vi "RT_Control_Adrian_ForceBalance.vi"(11 "Parameters":T1={"N_chan"=0, "Input Rate (Hz)"=0.0, "Acq Time (s)"=0.0, "NumOfWarmupIters"=0, "Size fifo"=0, "Period NCL (ms)"=0, "Timeout fifo Read"=0, "Size Sent Array"=0, "Output offsets"=[], "Input offsets"=[0.0, 0.0, 0.0, 0.0, 0.0, 0.0, 0.0, 0.0]}) -> (0 "error out":errorcluster, 1 "Total Iterations":i64, 2 "Delayed Cycles":dbl)   [LabVIEW 2021]
uses:
  parametersRT.ctl
  <vilib>/DAQmx/write.llb/DAQmx Write (Analog 1D DBL NChan 1Samp).vi
  <vilib>/DAQmx/read.llb/DAQmx Read (Analog 1D DBL NChan 1Samp).vi
  <vilib>/Analysis/baseanly.llb/A x Vector.vi
  <vilib>/DAQmx/configure/timing.llb/DAQmx Timing (Sample Clock).vi
  <vilib>/DAQmx/miscellaneous.llb/DAQmx Fill In Error Info.vi
  <resource>/objmgr/daqmx.rc
  <vilib>/Analysis/NI_AALBase.lvlib
panel:
  in  "source 2":tag
  in  "source":tag
  out "coerced(x)":dbl[](array[numeric])
  out "A x Vector":dbl[](array[numeric]) format="%.2f"
  in  "Unbias":bool
  out "Bias Voltages":dbl[][](array[numeric])=[[-0.0710179470114859, -0.17463349299050945, -0.11016159714741332, 0.026018829634351103, 0.12897648926553976, 0.08259620236774425]]
  out "Bias Vector":dbl[](array[numeric])=[-0.0710179470114859, -0.17463349299050945, -0.11016159714741332, 0.026018829634351103, 0.12897648926553976, 0.08259620236774425]
  in  "Bias":bool
  out "Voltages":dbl[][](array[numeric])=[[-0.07200476171213811, -0.17430455474177844, -0.11114841186574954, 0.027005644288728526, 0.12535816905124034, 0.08062257311350753], [-0.07233369994578917, -0.17397561649309423, -0.11147735010529275, 0.027334582506747616, 0.1263449836558195, 0.08160938774087402], [-0.0716758234785372, -0.17463349299050945, -0.11147735010529275, 0.026676706070656076, 0.1260160454543497, 0.08062257311350753], [-0.07200476171213811, -0.1749624312392873, -0.1118062883448848, 0.026676706070656076, 0.1256871072528233, 0.08029363490427514], [-0.07200476171213811, -0.17430455474177844, -0.11213522658452575, 0.026676706070656076, 0.12535816905124034, 0.08029363490427514], [-0.07233369994578917, -0.1749624312392873, -0.11147735010529275, 0.027334582506747616, 0.1260160454543497, 0.08062257311350753], [-0.07200476171213811, -0.17397561649309423, -0.11147735010529275, 0.027005644288728526, 0.1260160454543497, 0.08029363490427514], [-0.07200476171213811, -0.17463349299050945, -0.1118062883448848, 0.027005644288728526, 0.1260160454543497, 0.08062257311350753], [-0.07233369994578917, -0.17397561649309423, -0.11114841186574954, 0.027334582506747616, 0.1263449836558195, 0.08062257311350753], [-0.07233369994578917, -0.17463349299050945, -0.1118062883448848, 0.026676706070656076, 0.1256871072528233, 0.08029363490427514], [-0.07200476171213811, -0.17463349299050945, -0.11213522658452575, 0.027334582506747616, 0.1256871072528233, 0.08062257311350753], [-0.07233369994578917, -0.17463349299050945, -0.1118062883448848, 0.027005644288728526, 0.1256871072528233, 0.08029363490427514], [-0.07200476171213811, -0.17463349299050945, -0.1118062883448848, 0.027334582506747616, 0.1260160454543497, 0.08029363490427514], [-0.0716758234785372, -0.17430455474177844, -0.11147735010529275, 0.027334582506747616, 0.1263449836558195, 0.08128044953180698], [-0.07200476171213811, -0.17463349299050945, -0.11114841186574954, 0.027005644288728526, 0.1263449836558195, 0.08029363490427514], [-0.07266263817949037, -0.17430455474177844, -0.11213522658452575, 0.027005644288728526, 0.1256871072528233, 0.08029363490427514], [-0.07233369994578917, -0.17463349299050945, -0.1118062883448848, 0.027334582506747616, 0.1263449836558195, 0.08128044953180698], [-0.07200476171213811, -0.17397561649309423, -0.1118062883448848, 0.026676706070656076, 0.1260160454543497, 0.08029363490427514], [-0.07233369994578917, -0.17397561649309423, -0.11147735010529275, 0.027334582506747616, 0.1263449836558195, 0.08128044953180698], [-0.0716758234785372, -0.17397561649309423, -0.11147735010529275, 0.027334582506747616, 0.1256871072528233, 0.08029363490427514], [-0.07200476171213811, -0.17430455474177844, -0.1118062883448848, 0.027334582506747616, 0.1263449836558195, 0.08095151132268481], [-0.07266263817949037, -0.17463349299050945, -0.1118062883448848, 0.026676706070656076, 0.1260160454543497, 0.08029363490427514], [-0.07200476171213811, -0.1736466782444569, -0.1118062883448848, 0.027005644288728526, 0.12535816905124034, 0.08095151132268481], [-0.07233369994578917, -0.1749624312392873, -0.11147735010529275, 0.027005644288728526, 0.1263449836558195, 0.08062257311350753], [-0.07200476171213811, -0.1736466782444569, -0.11114841186574954, 0.02766352072471333, 0.1263449836558195, 0.08062257311350753], [-0.07200476171213811, -0.17463349299050945, -0.1118062883448848, 0.027005644288728526, 0.1256871072528233, 0.08029363490427514], [-0.07266263817949037, -0.17430455474177844, -0.11213522658452575, 0.027334582506747616, 0.1260160454543497, 0.08062257311350753], [-0.07200476171213811, -0.17430455474177844, -0.11147735010529275, 0.02766352072471333, 0.1263449836558195, 0.08062257311350753], [-0.07200476171213811, -0.1749624312392873, -0.11213522658452575, 0.027334582506747616, 0.1260160454543497, 0.08062257311350753], [-0.07233369994578917, -0.17430455474177844, -0.11147735010529275, 0.027334582506747616, 0.1260160454543497, 0.08029363490427514], [-0.07233369994578917, -0.17397561649309423, -0.1118062883448848, 0.027334582506747616, 0.1263449836558195, 0.08062257311350753], [-0.0716758234785372, -0.17397561649309423, -0.11213522658452575, 0.027334582506747616, 0.1260160454543497, 0.07996469669498764], [-0.07266263817949037, -0.17430455474177844, -0.1118062883448848, 0.02766352072471333, 0.1263449836558195, 0.08062257311350753], [-0.07266263817949037, -0.17430455474177844, -0.1118062883448848, 0.027334582506747616, 0.1256871072528233, 0.08029363490427514], [-0.07200476171213811, -0.17463349299050945, -0.1118062883448848, 0.026676706070656076, 0.12535816905124034, 0.07963575848564507], [-0.07233369994578917, -0.17397561649309423, -0.11114841186574954, 0.02766352072471333, 0.1263449836558195, 0.08062257311350753], [-0.07266263817949037, -0.1749624312392873, -0.11213522658452575, 0.026676706070656076, 0.12535816905124034, 0.07963575848564507], [-0.07233369994578917, -0.17463349299050945, -0.1118062883448848, 0.027005644288728526, 0.1256871072528233, 0.07996469669498764], [-0.07299157641324171, -0.17463349299050945, -0.11213522658452575, 0.026676706070656076, 0.1260160454543497, 0.08029363490427514], [-0.07233369994578917, -0.17430455474177844, -0.11147735010529275, 0.027334582506747616, 0.12667392185723272, 0.08095151132268481], [-0.07200476171213811, -0.1736466782444569, -0.11147735010529275, 0.02766352072471333, 0.1263449836558195, 0.08062257311350753], [-0.07233369994578917, -0.17397561649309423, -0.1118062883448848, 0.026676706070656076, 0.1260160454543497, 0.07996469669498764], [-0.07233369994578917, -0.17463349299050945, -0.11213522658452575, 0.027005644288728526, 0.1260160454543497, 0.08029363490427514], [-0.07200476171213811, -0.17331773999586642, -0.11081947362625524, 0.02766352072471333, 0.12667392185723272, 0.08095151132268481], [-0.07233369994578917, -0.17397561649309423, -0.1118062883448848, 0.02766352072471333, 0.1260160454543497, 0.08029363490427514], [-0.07266263817949037, -0.17463349299050945, -0.11213522658452575, 0.02766352072471333, 0.1260160454543497, 0.08128044953180698], [-0.07200476171213811, -0.17397561649309423, -0.11147735010529275, 0.02766352072471333, 0.1263449836558195, 0.08095151132268481], [-0.07200476171213811, -0.17430455474177844, -0.1118062883448848, 0.027334582506747616, 0.1263449836558195, 0.08095151132268481], [-0.0716758234785372, -0.17463349299050945, -0.1118062883448848, 0.027005644288728526, 0.1263449836558195, 0.08095151132268481], [-0.07200476171213811, -0.17397561649309423, -0.1118062883448848, 0.027005644288728526, 0.1256871072528233, 0.08029363490427514], [-0.07233369994578917, -0.17430455474177844, -0.11147735010529275, 0.027334582506747616, 0.1263449836558195, 0.08095151132268481], [-0.0716758234785372, -0.1736466782444569, -0.11114841186574954, 0.027992458942625646, 0.12667392185723272, 0.08095151132268481], [-0.07200476171213811, -0.17397561649309423, -0.1118062883448848, 0.027334582506747616, 0.1263449836558195, 0.08029363490427514], [-0.07200476171213811, -0.17397561649309423, -0.11114841186574954, 0.027334582506747616, 0.1263449836558195, 0.08029363490427514], [-0.07233369994578917, -0.17397561649309423, -0.1118062883448848, 0.027334582506747616, 0.1260160454543497, 0.08029363490427514], [-0.07266263817949037, -0.17430455474177844, -0.11213522658452575, 0.026676706070656076, 0.1260160454543497, 0.08029363490427514], [-0.07233369994578917, -0.17397561649309423, -0.11213522658452575, 0.027334582506747616, 0.1263449836558195, 0.08062257311350753], [-0.07233369994578917, -0.17463349299050945, -0.11213522658452575, 0.027334582506747616, 0.1260160454543497, 0.08029363490427514], [-0.07200476171213811, -0.17331773999586642, -0.11147735010529275, 0.027334582506747616, 0.1263449836558195, 0.08029363490427514], [-0.07233369994578917, -0.1749624312392873, -0.11213522658452575, 0.026676706070656076, 0.1260160454543497, 0.08029363490427514], [-0.07233369994578917, -0.17463349299050945, -0.1118062883448848, 0.027005644288728526, 0.1260160454543497, 0.08029363490427514], [-0.07233369994578917, -0.17397561649309423, -0.1118062883448848, 0.027334582506747616, 0.12667392185723272, 0.08062257311350753], [-0.07200476171213811, -0.17430455474177844, -0.11147735010529275, 0.027334582506747616, 0.1260160454543497, 0.07996469669498764], [-0.07233369994578917, -0.17430455474177844, -0.1118062883448848, 0.027334582506747616, 0.12667392185723272, 0.08095151132268481], [-0.0716758234785372, -0.17430455474177844, -0.11147735010529275, 0.026676706070656076, 0.1263449836558195, 0.08029363490427514], [-0.07266263817949037, -0.17430455474177844, -0.11147735010529275, 0.027005644288728526, 0.1263449836558195, 0.07996469669498764], [-0.07266263817949037, -0.1749624312392873, -0.11246416482421552, 0.026676706070656076, 0.1263449836558195, 0.08029363490427514], [-0.07266263817949037, -0.17397561649309423, -0.1118062883448848, 0.027334582506747616, 0.1263449836558195, 0.08029363490427514], [-0.0716758234785372, -0.1736466782444569, -0.11147735010529275, 0.02766352072471333, 0.1263449836558195, 0.08062257311350753], [-0.07233369994578917, -0.17397561649309423, -0.1118062883448848, 0.027334582506747616, 0.1263449836558195, 0.08095151132268481], [-0.07233369994578917, -0.17430455474177844, -0.1118062883448848, 0.027334582506747616, 0.1260160454543497, 0.08062257311350753], [-0.0716758234785372, -0.17331773999586642, -0.11081947362625524, 0.027992458942625646, 0.12700286005858935, 0.08062257311350753], [-0.07233369994578917, -0.17397561649309423, -0.11213522658452575, 0.027005644288728526, 0.1263449836558195, 0.08029363490427514], [-0.07233369994578917, -0.17463349299050945, -0.11147735010529275, 0.027005644288728526, 0.1260160454543497, 0.08029363490427514], [-0.07266263817949037, -0.1736466782444569, -0.11147735010529275, 0.02766352072471333, 0.12667392185723272, 0.08029363490427514], [-0.07200476171213811, -0.17463349299050945, -0.11213522658452575, 0.026676706070656076, 0.1260160454543497, 0.07996469669498764], [-0.07266263817949037, -0.17430455474177844, -0.11213522658452575, 0.027005644288728526, 0.1263449836558195, 0.08062257311350753], [-0.07200476171213811, -0.17397561649309423, -0.11147735010529275, 0.02766352072471333, 0.1263449836558195, 0.08062257311350753], [-0.07200476171213811, -0.17397561649309423, -0.1118062883448848, 0.027005644288728526, 0.1263449836558195, 0.08029363490427514], [-0.07233369994578917, -0.17430455474177844, -0.11213522658452575, 0.027005644288728526, 0.1263449836558195, 0.08062257311350753], [-0.07233369994578917, -0.1736466782444569, -0.11114841186574954, 0.027334582506747616, 0.12667392185723272, 0.08062257311350753], [-0.07233369994578917, -0.17430455474177844, -0.1118062883448848, 0.027334582506747616, 0.1260160454543497, 0.08029363490427514], [-0.07266263817949037, -0.17529136948811197, -0.11279310306395414, 0.026676706070656076, 0.1263449836558195, 0.08029363490427514], [-0.07233369994578917, -0.17397561649309423, -0.11147735010529275, 0.027005644288728526, 0.12667392185723272, 0.08062257311350753], [-0.07200476171213811, -0.17430455474177844, -0.1118062883448848, 0.027334582506747616, 0.1263449836558195, 0.07996469669498764], [-0.07233369994578917, -0.17463349299050945, -0.11246416482421552, 0.027005644288728526, 0.1256871072528233, 0.07996469669498764], [-0.07266263817949037, -0.17430455474177844, -0.1118062883448848, 0.026676706070656076, 0.1260160454543497, 0.07996469669498764], [-0.07266263817949037, -0.17463349299050945, -0.1118062883448848, 0.027005644288728526, 0.1260160454543497, 0.08062257311350753], [-0.07266263817949037, -0.17397561649309423, -0.1118062883448848, 0.02766352072471333, 0.1263449836558195, 0.07996469669498764], [-0.07233369994578917, -0.17463349299050945, -0.1118062883448848, 0.027005644288728526, 0.1260160454543497, 0.08062257311350753], [-0.0716758234785372, -0.17397561649309423, -0.11114841186574954, 0.02766352072471333, 0.12667392185723272, 0.08095151132268481], [-0.07200476171213811, -0.17430455474177844, -0.11147735010529275, 0.027005644288728526, 0.1260160454543497, 0.08029363490427514], [-0.07200476171213811, -0.17397561649309423, -0.11114841186574954, 0.027992458942625646, 0.12700286005858935, 0.08128044953180698], [-0.07134688524498646, -0.17397561649309423, -0.1118062883448848, 0.027005644288728526, 0.1263449836558195, 0.07996469669498764], [-0.07266263817949037, -0.17463349299050945, -0.11213522658452575, 0.026676706070656076, 0.1256871072528233, 0.07996469669498764], [-0.07266263817949037, -0.17430455474177844, -0.11147735010529275, 0.027334582506747616, 0.12667392185723272, 0.08062257311350753], [-0.0716758234785372, -0.17463349299050945, -0.1118062883448848, 0.026676706070656076, 0.12667392185723272, 0.08029363490427514], [-0.07233369994578917, -0.17397561649309423, -0.1118062883448848, 0.027334582506747616, 0.1263449836558195, 0.08062257311350753], [-0.07233369994578917, -0.17463349299050945, -0.1118062883448848, 0.027005644288728526, 0.1260160454543497, 0.08029363490427514], [-0.07233369994578917, -0.17397561649309423, -0.11213522658452575, 0.027334582506747616, 0.1263449836558195, 0.08062257311350753]]
  out "output array":dbl[](array[numeric])
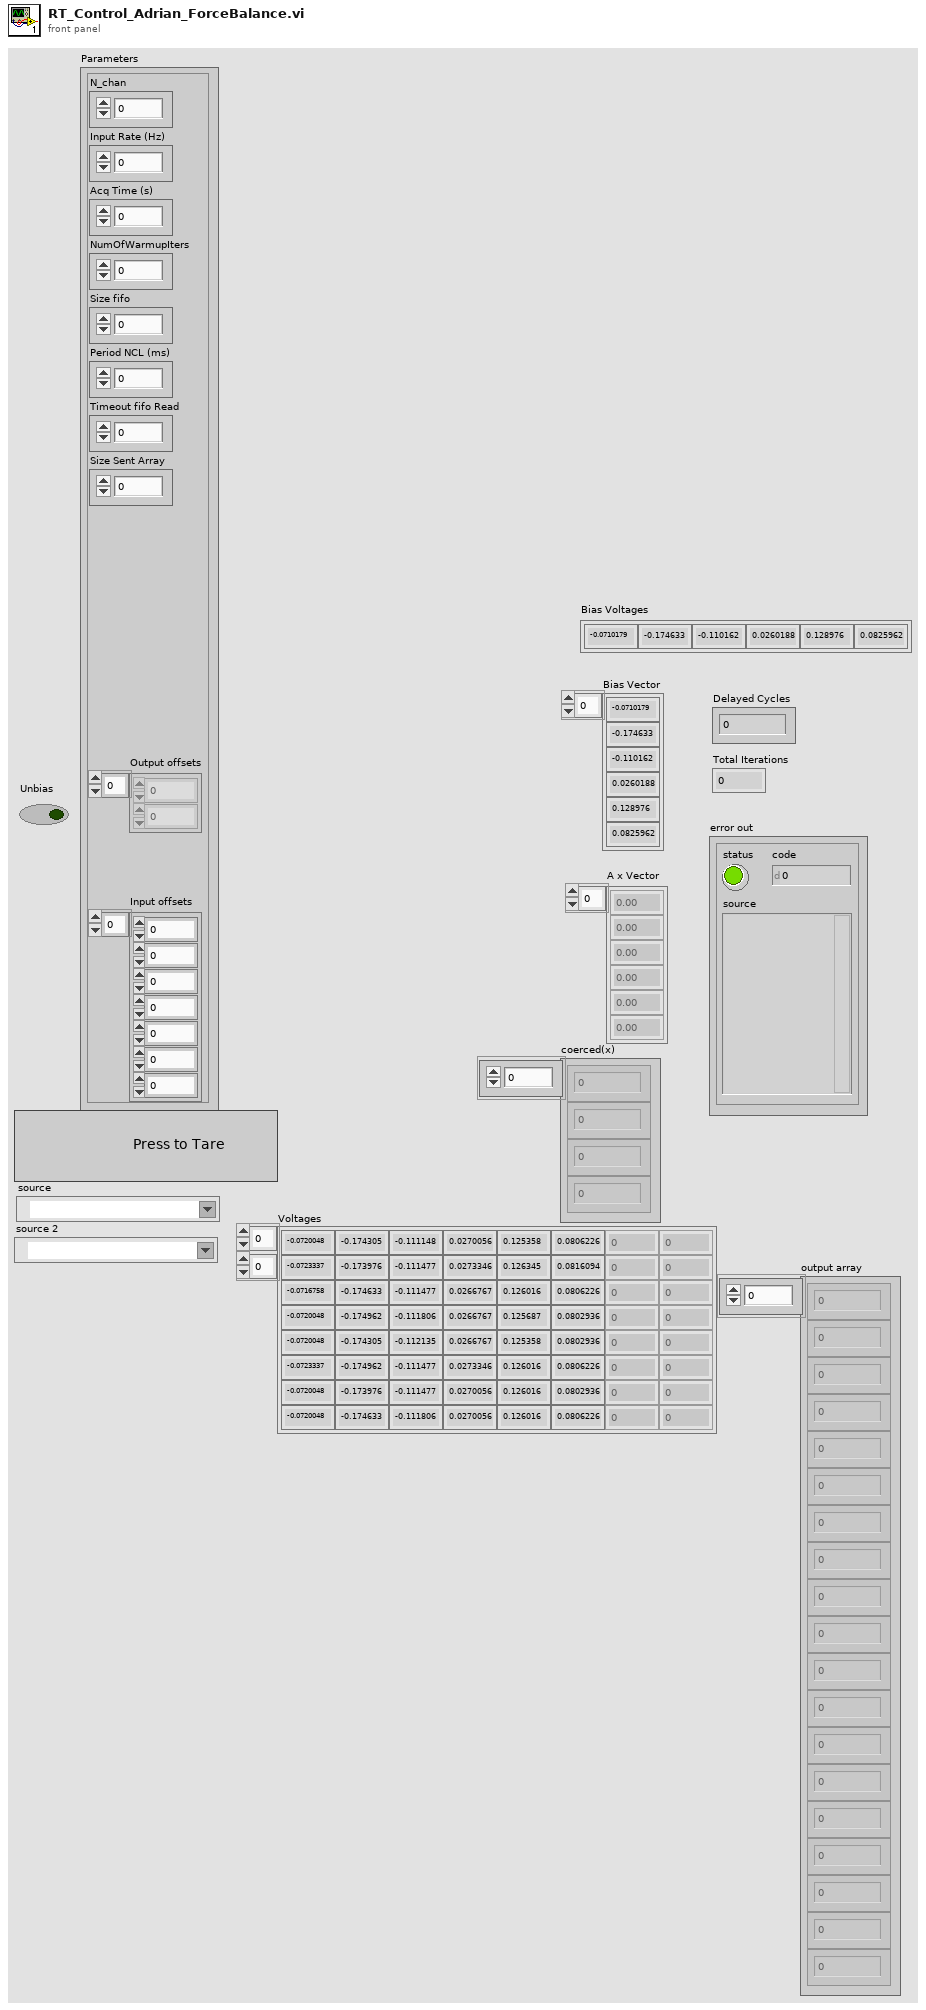
[diagram p1: front panel]
types:
  T1 = typedef "parametersRT.ctl" = cluster{"N_chan":u32, "Input Rate (Hz)":dbl, "Acq Time (s)":dbl, "NumOfWarmupIters":u32, "Size fifo":u32, "Period NCL (ms)":i64, "Timeout fifo Read":i32, "Size Sent Array":i32, "Output offsets":dbl[], "Input offsets":dbl[]}
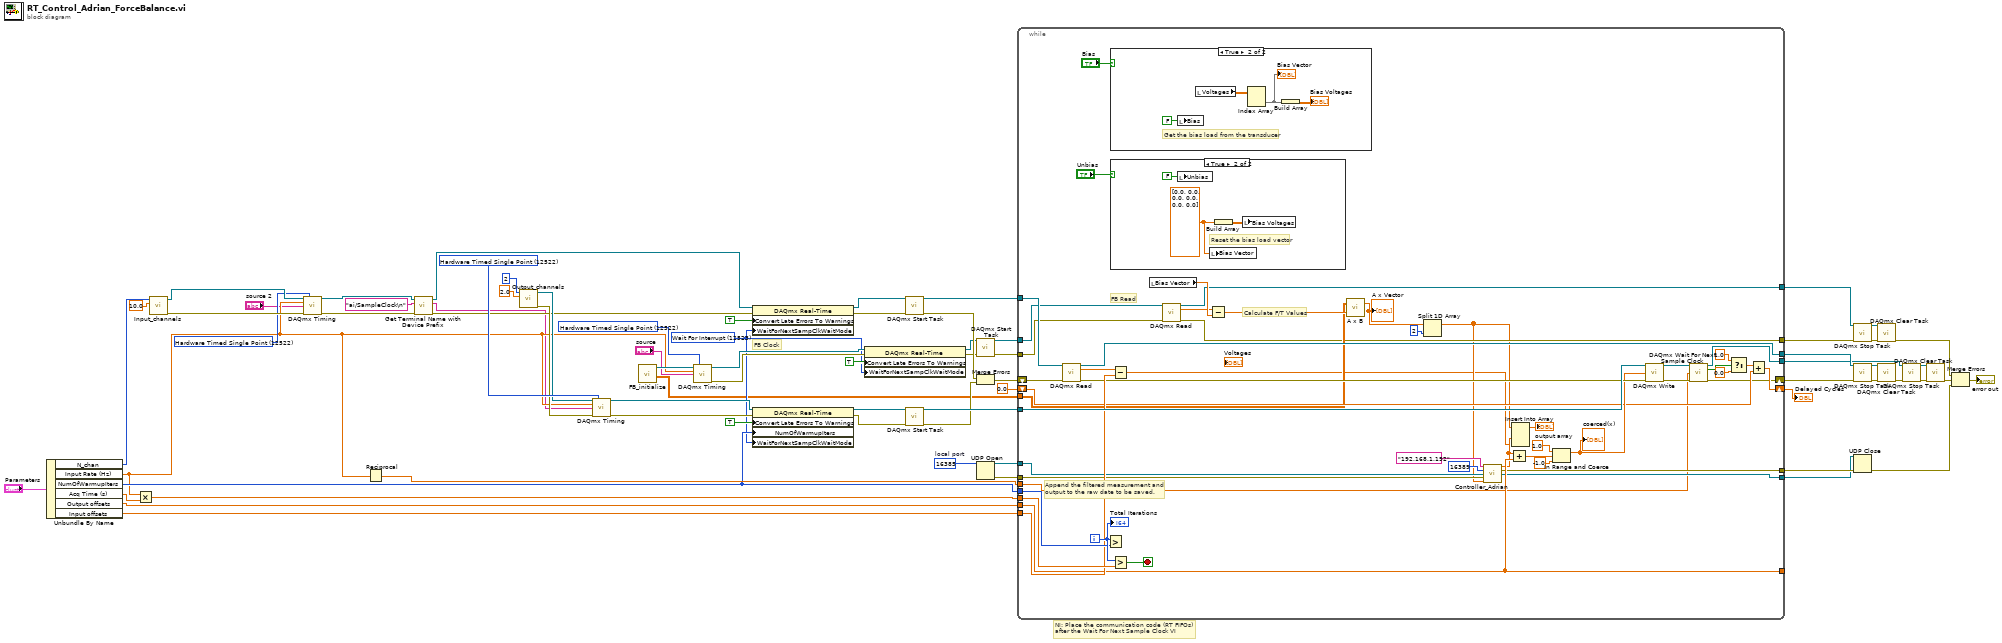
[diagram p0: block diagram]
diagram:
  w31 = 12522 items=["Finite Samples"=10178, "Continuous Samples"=10123, "Hardware Timed Single Point"=12522] ("sample mode")
  w42 = u16 16385  # local port
  w49 = 12522 items=["Finite Samples"=10178, "Continuous Samples"=10123, "Hardware Timed Single Point"=12522] ("sample mode")
  w26 = 12523 items=["Wait For Interrupt"=12523, "Poll"=12524, "Yield"=12525] ("WaitForNextSampClkWaitMode")
  w72 = 12522 items=["Finite Samples"=10178, "Continuous Samples"=10123, "Hardware Timed Single Point"=12522] ("sample mode")
  # "FB Clock"
  # "NI: Place the communication code (RT FIFOs) \nafter the Wait For Next Sample Clock VI"
  n1 = Unbundle By Name("Parameters") -> ("N_chan"=w58:u32, "Input Rate (Hz)"=w25:dbl, "NumOfWarmupIters"=w59:u32, "Acq Time (s)"=w66:dbl, "Output offsets"=w57:dbl[], "Input offsets"=w56:dbl[])
  n2 = Multiply(x=w25, y=w66) -> (x*y=w36:dbl)
  n3 = call "Input_channels.vi"("Range"=10.0, "nchan"=w58) -> ("error out"=w51:errorcluster, "Refnum out"=w50:refnum<k21>)  [unwired: 8 in]
  n4 = call-poly <vilib>:"DAQmx Timing.vi"("task/channels in"=w50, "sample mode"=w49, "rate"=w25, "source"="source 2", "error in"=w51) -> ("task out"=w18:refnum<k21>, "error out"=w16:errorcluster)  [unwired: 9 in]
  n5 = Reciprocal(x=w25) -> (1/x=w71:dbl)
  n6 = call "Get Terminal Name with Device Prefix.vi"("error in (no error)"=w16, "Local Terminal Name"="ai/SampleClock\n", "task/channels in"=w18) -> ("error out"=w15:errorcluster, "Terminal Name with Device Prefix"=w14:tag, "task out"=w17:refnum<k21>)  [unwired: 6 in]
  n7 = call "Output_channels.vi"("Range"=2.0 ("Maximum Value"), "nchan"=2) -> ("error out"=w63:errorcluster, "Refnum out"=w62:refnum<k21>)  [unwired: 8 in]
  n8 = call-poly <vilib>:"DAQmx Timing.vi"("task/channels in"=w62, "sample mode"=w72, "rate"=w25, "source"=w14, "error in"=w63) -> ("task out"=w70:refnum<k21>, "error out"=w69:errorcluster)  [unwired: 9 in]
  n9 = call "FB_initialize.vi"() -> ("Transformed Calibration Matrix"=w22:dbl[][], "FB out"=w27:refnum<k21>)  [unwired: 9 in, 1 out]
  n10 = call-poly <vilib>:"DAQmx Timing.vi"("task/channels in"=w27, "sample mode"=w31, "rate"=w25, "source"="source") -> ("task out"=w33:refnum<k21>, "error out"=w32:errorcluster)  [unwired: 10 in]
  n11 = property class="DAQmx Real-Time"(reference=w17, error in=w15, "Convert Late Errors To Warnings"=TRUE, "WaitForNextSampClkWaitMode"=w26) -> (reference out=w46:refnum<k21>, error out=w45:errorcluster)
  n12 = property class="DAQmx Real-Time"(reference=w70, error in=w69, "Convert Late Errors To Warnings"=TRUE, "NumOfWarmupIters"=w59, "WaitForNextSampClkWaitMode"=w26) -> (reference out=w67:refnum<k21>, error out=w53:errorcluster)
  n13 = property class="DAQmx Real-Time"(reference=w33, error in=w32, "Convert Late Errors To Warnings"=TRUE ("ConvLateErrorsToWarnings"), "WaitForNextSampClkWaitMode"=w26) -> (reference out=w28:refnum<k21>, error out=w29:errorcluster)
  n14 = call <vilib>:"DAQmx Start Task.vi"("task/channels in"=w46, "error in"=w45) -> ("task out"=w65:refnum<k21>, "error out"=w44:errorcluster)  [unwired: 12 in]
  n15 = call <vilib>:"DAQmx Start Task.vi"("task/channels in"=w67, "error in"=w53) -> ("task out"=w64:refnum<k21>, "error out"=w52:errorcluster)  [unwired: 12 in]
  n16 = call <vilib>:"DAQmx Start Task.vi"("task/channels in"=w28, "error in"=w29) -> ("task out"=w24:refnum<k21>, "error out"=w23:errorcluster)  [unwired: 12 in]
  n17 = Merge Errors(w44, w52) -> (w43:errorcluster)
  n18 = UDP Open(11:w42) -> (port=w40:refnum<k16>, 0:w41:errorcluster)  [unwired: 4 in, 1 out]
  n19 = while {
    shift-right: [w74] -> w7
    shift-left: w43 -> [w109]
    shift-right: [w119] -> w73
    shift-left: 0.0 ("f") -> [w97]
    tunnel: w71 -> [w75]
    tunnel: w36 -> [w117]
    tunnel: w64 -> [w116]
    tunnel: [w110] -> w6
    tunnel: w65 -> [w111]
    tunnel: [w77] -> w2
    tunnel: w59 -> [w113]
    tunnel: w57 -> [w105]
    tunnel: [w105] -> _
    tunnel: w56 -> [w112]
    tunnel: w41 -> [w103]
    tunnel: w40 -> [w102]
    tunnel: [w101] -> w39
    tunnel: [w100] -> w38
    tunnel: w24 -> [w95]
    tunnel: w23 -> [w94]
    tunnel: w22 -> [w88]
    tunnel: [w87] -> w12
    tunnel: [w86] -> w10
    i -> [w114]
    stop <- w118 stop-if-true
    # "Calculate F/T Values"
    # "FB Read"
    # "Append the filtered measurement and \noutput to the raw date to be saved."
    n20 = call-poly <vilib>:"DAQmx Read.vi"("task/channels in"=w111, "error in"=w109) -> ("task out"=w110:refnum<k21>, "data"=w96:dbl[], "error out"=w108:errorcluster)  [unwired: 11 in]
    n21 = Greater?(x=w114, y=w113) -> ()  [unwired: 1 out]
    n22 = case shown="True" "Bias" {
      frame False {
      }
      frame True {
        # "Get the bias load from the transducer"
        n23 = local write "Bias"(FALSE) -> ()
        n24 = local read "Voltages"() -> (w129:dbl[][])
        n25 = Index Array(array=w129) -> (element=w126:dbl[])  [unwired: 2 in]
        "Bias Vector" <- w126
        n26 = Build Array(w126) -> (→"Bias Voltages":dbl[][])
      }
    }
    n27 = case shown="True" "Unbias" {
      frame False {
      }
      frame True {
        w124 = dbl[] [0.0, 0.0, 0.0, 0.0, 0.0, 0.0]
        # "Reset the bias load vector"
        n28 = local write "Unbias"(FALSE) -> ()
        n29 = local write "Bias Vector"(w124) -> ()
        n30 = Build Array(w124) -> (w123:dbl[][])
        n31 = local write "Bias Voltages"(w123) -> ()
      }
    }
    n32 = Subtract(x=w96, y=w112) -> (x-y=w80:dbl[])
    n33 = Greater?(x=w114, y=w117) -> (0:w118:bool)
    n34 = local read "Bias Vector"() -> (w91:dbl[])
    n35 = call-poly <vilib>:"DAQmx Read.vi"("task/channels in"=w95, "error in"=w94) -> ("task out"=w87:refnum<k21>, "data"=w89:dbl[], "error out"=w86:errorcluster)  [unwired: 11 in]
    n36 = Subtract(x=w89, y=w91) -> (x-y=w90:dbl[])
    n37 = call-poly <vilib>:"A x B.vi"("Vector"=w90, "A"=w88) -> ("A x Vector"=w84:dbl[])  [unwired: 1 out]
    "A x Vector" <- w84
    n38 = Split 1D Array(array=w84, index=2) -> (first subarray=w83:dbl[])  [unwired: 1 out]
    n39 = call "Controller_Adrian.vi"("name 2"="192.168.1.192", "port or service name"=u16 16389, "connection ID"=w102, "error in (no error)"=w103, "x"=w83) -> ("*(type *) &x"=w81:dbl[], "error out"=w101:errorcluster, "connection ID out"=w100:refnum<k16>)  [unwired: 8 in]
    n40 = Add(x=w81, y=w105) -> (x+y=w82:dbl[])
    n41 = Insert Into Array(array=w83, new element #1=w81, new element #2=w80) -> (→"output array":dbl[])  [unwired: 1 in]
    n42 = In Range and Coerce(upper limit=1.0, x=w82, lower limit=-1.0) -> (coerced(x)=w104:dbl[])  [unwired: 1 out]
    "coerced(x)" <- w104
    n43 = call-poly <vilib>:"DAQmx Write.vi"("task/channels in"=w116, "data"=w104, "error in"=w108) -> ("task out"=w78:refnum<k21>, "error out"=w79:errorcluster)  [unwired: 10 in, 1 out]
    n44 = call <vilib>:"DAQmx Wait For Next Sample Clock.vi"("task/channels in"=w78, "timeout (sec)"=w75, "error in"=w79) -> ("task out"=w77:refnum<k21>, "is late?"=w76:bool, "error out"=w74:errorcluster)  [unwired: 10 in]
    n45 = Select(t=1.0, s=w76, f=0.0) -> (s? t:f=w120:dbl)
    n46 = Add(x=w120, y=w97) -> (x+y=w119:dbl)
    "Total Iterations" <- w114
  }
  "Delayed Cycles" <- w73
  n47 = call <vilib>:"DAQmx Stop Task.vi"("task/channels in"=w12, "error in"=w10) -> ("task out"=w11:refnum<k21>, "error out"=w9:errorcluster)  [unwired: 12 in]
  n48 = call <vilib>:"DAQmx Stop Task.vi"("task/channels in"=w6, "error in"=w7) -> ("task out"=w5:refnum<k21>, "error out"=w8:errorcluster)  [unwired: 12 in]
  n49 = UDP Close(connection ID=w38, 8:w39) -> (error out=w37:errorcluster)  [unwired: 1 out]
  n50 = call <vilib>:"DAQmx Clear Task.vi"("task in"=w11, "error in"=w9) -> ("error out"=w21:errorcluster)  [unwired: 13 in]
  n51 = call <vilib>:"DAQmx Clear Task.vi"("task in"=w5, "error in"=w8) -> ("error out"=w4:errorcluster)  [unwired: 13 in]
  n52 = call <vilib>:"DAQmx Stop Task.vi"("task/channels in"=w2, "error in"=w4) -> ("task out"=w1:refnum<k21>, "error out"=w3:errorcluster)  [unwired: 12 in]
  n53 = call <vilib>:"DAQmx Clear Task.vi"("task in"=w1, "error in"=w3) -> ("error out"=w55:errorcluster)  [unwired: 13 in]
  n54 = Merge Errors(w21, w55, w37) -> (→"error out":errorcluster)
